vi "HFRR ADV v06 new software.vi"() -> ()   [LabVIEW 2025] (continued)
                  n3117 = local write "S 59"(w4151) -> ()
                }
                frame 59 {
                  n3118 = local write "S 60"(w4152) -> ()
                }
                frame 60 {
                  n3119 = local write "S 62"(w4153) -> ()
                }
                frame 61 {
                  n3120 = local write "S 63"(w4154) -> ()
                }
                frame 62 {
                  n3121 = local write "S 64"(w4155) -> ()
                }
                frame 63 {
                  n3122 = local write "S 65"(w4156) -> ()
                }
                frame 64 {
                  n3123 = local write "S 66"(w4157) -> ()
                }
                frame 65 {
                  n3124 = local write "S 67"(w4158) -> ()
                }
                frame 66 {
                  n3125 = local write "S 68"(w4159) -> ()
                }
                frame 67 {
                  n3126 = local write "S 69"(w4160) -> ()
                }
                frame 68 {
                  n3127 = local write "S 70"(w4161) -> ()
                }
                frame 69 {
                  n3128 = local write "S 71"(w4162) -> ()
                }
                frame 70 {
                  n3129 = local write "S 72"(w4163) -> ()
                }
                frame 71 {
                  n3130 = local write "S 73"(w4164) -> ()
                }
                frame 72 {
                  n3131 = local write "S 74"(w4165) -> ()
                }
                frame 73 {
                  n3132 = local write "S 75"(w4166) -> ()
                }
                frame 74 {
                  n3133 = local write "S 76"(w4167) -> ()
                }
                frame 75 {
                  n3134 = local write "S 77"(w4168) -> ()
                }
                frame 76 {
                  n3135 = local write "S 78"(w4169) -> ()
                }
                frame 77 {
                  n3136 = local write "S 79"(w4170) -> ()
                }
                frame 79 {
                  n3137 = property on="Sample Temperature ( °C )" class="XYGraph (strict)"("Y Scale.Name Label.Text"=w4171) -> ()  [unwired: 2 in, 2 out]
                }
                frame 80 {
                  n3138 = local write "S 81"(w4172) -> ()
                  n3139 = property on="Humidity ( %RH )" class="XYGraph (strict)"("Y Scale.Name Label.Text"=w4172) -> ()  [unwired: 2 in, 2 out]
                }
                frame 78 {
                  n3140 = property on="Air Temperature  ( °C )" class="XYGraph (strict)"("X Scale.Name Label.Text"=w4173) -> ()  [unwired: 2 in, 2 out]
                  n3141 = property on="Humidity ( %RH )" class="XYGraph (strict)"("X Scale.Name Label.Text"=w4173) -> ()  [unwired: 2 in, 2 out]
                  n3142 = property on="Sample Temperature ( °C )" class="XYGraph (strict)"("X Scale.Name Label.Text"=w4173) -> ()  [unwired: 2 in, 2 out]
                  n3143 = property on="Coefficient Of Friction" class="XYGraph (strict)"("X Scale.Name Label.Text"=w4173) -> ()  [unwired: 2 in, 2 out]
                }
                frame 81 {
                  n3144 = property on="Air Temperature  ( °C )" class="XYGraph (strict)"("Y Scale.Name Label.Text"=w4174) -> ()  [unwired: 2 in, 2 out]
                }
                frame 82 {
                  n3145 = local write "S 84"(w4175) -> ()
                }
                frame 83 {
                  n3146 = local write "S 85"(w4176) -> ()
                }
                frame 84 {
                  n3147 = local write "S 86"(w4177) -> ()
                }
                frame 85 {
                  n3148 = local write "S 87"(w4178) -> ()
                }
                frame 86 {
                  n3149 = local write "S 88"(w4179) -> ()
                }
                frame 87 {
                }
                frame 88 {
                  n3150 = local write "S 90"(w4181) -> ()
                }
                frame 89 {
                  n3151 = local write "S 91"(w4182) -> ()
                }
                frame 90 {
                  n3152 = local write "S 92"(w4183) -> ()
                }
                frame 91 {
                  n3153 = local write "S 93"(w4184) -> ()
                }
                frame 92 {
                  n3154 = local write "S 94"(w4185) -> ()
                }
                frame 93 {
                  n3155 = local write "S 95"(w4186) -> ()
                }
                frame 94 {
                  n3156 = local write "S 96"(w4187) -> ()
                }
                frame 95 {
                  n3157 = local write "S 97"(w4188) -> ()
                }
                frame 96 {
                  n3158 = local write "S 98"(w4189) -> ()
                }
                frame 97 {
                  n3159 = local write "S 99"(w4190) -> ()
                }
                frame 98 {
                  n3160 = local write "S 100"(w4191) -> ()
                }
                frame 99 {
                  n3161 = local write "S 101"(w4192) -> ()
                }
                frame 100 {
                  n3162 = local write "S 102"(w4193) -> ()
                }
                frame 101 {
                  n3163 = local write "S 103"(w4194) -> ()
                }
                frame 102 {
                  n3164 = local write "S 104"(w4195) -> ()
                }
                frame 103 {
                  n3165 = local write "S 105"(w4196) -> ()
                }
                frame 104 {
                  n3166 = local write "S 106"(w4197) -> ()
                }
                frame 105 {
                }
                frame 106 {
                  n3167 = property on="OK Button 17" class="Bool (strict)"("Boolean Text.Text"=w4198) -> ()  [unwired: 2 in, 2 out]
                }
                frame 107 {
                  n3168 = property on="OK Button 16" class="Bool (strict)"("Boolean Text.Text"=w4199) -> ()  [unwired: 2 in, 2 out]
                }
                frame 108 {
                  n3169 = property on="TITTLE" class="Str"("Caption.Text"=w4200) -> ()  [unwired: 2 in, 2 out]
                }
                frame 109 {
                  "String 30" <- w4201
                }
                frame 110 {
                  n3170 = property on="Test Date" class="Str"("Caption.Text"=w4202) -> ()  [unwired: 2 in, 2 out]
                  "String 31" <- w4202
                }
                frame 111 {
                  n3171 = property on="Sample ID" class="Str"("Caption.Text"=w4203) -> ()  [unwired: 2 in, 2 out]
                  "String 32" <- w4203
                }
                frame 112 {
                  n3172 = property on="Tested by" class="Str"("Caption.Text"=w4204) -> ()  [unwired: 2 in, 2 out]
                  "String 33" <- w4204
                }
                frame 113 {
                  n3173 = property on="System Configured Printers 2" class="Arr (strict)"("Caption.Text"=w4205) -> ()  [unwired: 2 in, 2 out]
                }
                frame 114 {
                  n3174 = property on="Selected Printer" class="Str"("Caption.Text"=w4206) -> ()  [unwired: 2 in, 2 out]
                }
                frame 115 {
                  n3175 = property on="Select Printer 3" class="DigNum (strict)"("Caption.Text"=w4207) -> ()  [unwired: 2 in, 2 out]
                }
                frame 116 {
                  n3176 = property on="Print" class="Bool (strict)"("Boolean Text.Text"=w4208) -> ()  [unwired: 2 in, 2 out]
                }
                frame 117 {
                  "String 41" <- w4209
                }
                frame 118 {
                  n3177 = property on="tested by" class="Str"("Caption.Text"=w4210) -> ()  [unwired: 2 in, 2 out]
                }
                frame 119 {
                }
                frame 120 {
                  n3178 = property on="Export" class="Bool (strict)"("Boolean Text.Text"=w4211) -> ()  [unwired: 2 in, 2 out]
                }
                frame 121 {
                  n3179 = property on="TEMP INTERCEPT:" class="DigNum (strict)"("Caption.Text"=w4212) -> ()  [unwired: 2 in, 2 out]
                }
                frame 122 {
                  n3180 = property on="AIR TEMP INTERCEPT:" class="DigNum (strict)"("Caption.Text"=w4213) -> ()  [unwired: 2 in, 2 out]
                }
                frame 123 {
                  n3181 = property on="Select File Type" class="Enum (strict)"("Caption.Text"=w4214) -> ()  [unwired: 2 in, 2 out]
                }
                frame 124 {
                  n3182 = property on="s.NO" class="Str"("Caption.Text"=w4215) -> ()  [unwired: 2 in, 2 out]
                  "String 45" <- w4215
                }
                frame 125 {
                  n3183 = property on="trip1 8" class="Bool (strict)"("Boolean Text.Text"=w4216) -> ()  [unwired: 2 in, 2 out]
                }
                frame 126, Default {
                }
              }
            }
          }
          frame #1 {
            w4224 = TRUE ("Visible")
            n3184 = local read "S 91"() -> (w4241:string)
            n3185 = local read "S 90"() -> (w4240:string)
            n3186 = local read "S 88"() -> (w4239:string)
            n3187 = property on="File Path" class="Path"("Caption.Text"=w4240) -> ()  [unwired: 2 in, 2 out]
            n3188 = property on="SrvM CP" class="Bool (strict)"("Boolean Text.Text"=w4239) -> ()  [unwired: 2 in, 2 out]
            n3189 = local read "S 71"() -> (w4234:string)
            n3190 = local read "S 86"() -> (w4236:string)
            n3191 = local read "S 85"() -> (w4237:string)
            n3192 = local read "S 87"() -> (w4235:string)
            n3193 = local read "S 84"() -> (w4238:string)
            n3194 = local read "S 103"() -> (w4223:string)
            n3195 = local read "S 104"() -> (w4222:string)
            n3196 = property on="ENTER THE NEW PASSWORD" class="Str"("Caption.Text"=w4235) -> ()  [unwired: 2 in, 2 out]
            n3197 = property on="Password" class="Str"("Caption.Text"=w4237) -> ()  [unwired: 2 in, 2 out]
            n3198 = property on="ENTER CURRENT PASSWORD" class="Str"("Caption.Text"=w4236) -> ()  [unwired: 2 in, 2 out]
            n3199 = property on="EDIT" class="Bool (strict)"("Boolean Text.Text"=w4234) -> ()  [unwired: 2 in, 2 out]
            n3200 = property on="SAVE" class="Bool (strict)"("Boolean Text.Text"=w4238) -> ()  [unwired: 2 in, 2 out]
            n3201 = Build Array(w4223, w4222) -> (w4221:string[])
            n3202 = property on="Heater Button" class="Bool (strict)"("Strings [4]"=w4221) -> ()  [unwired: 2 in, 2 out]
            n3203 = property on="CH-HUMIDITY WET" class="DigNum (strict)"("Caption.Size to Text?"=w4224) -> ()  [unwired: 2 in, 2 out]
            n3204 = property on="CH-HUMIDITY DRY" class="DigNum (strict)"("Caption.Size to Text?"=w4224) -> ()  [unwired: 2 in, 2 out]
            n3205 = property on="CH-POWER -" class="DigNum (strict)"("Caption.Size to Text?"=w4224) -> ()  [unwired: 2 in, 2 out]
            n3206 = property on="CH-HEATER" class="DigNum (strict)"("Caption.Size to Text?"=w4224) -> ()  [unwired: 2 in, 2 out]
            n3207 = property on="CH-POWER +" class="DigNum (strict)"("Caption.Size to Text?"=w4224) -> ()  [unwired: 2 in, 2 out]
            n3208 = local read "S 92"() -> (w4233:string)
            n3209 = local read "S 93"() -> (w4232:string)
            n3210 = local read "S 105"() -> (w4219:string)
            n3211 = local read "S 106"() -> (w4218:string)
            n3212 = Build Array(w4233, w4232) -> ()  [unwired: 1 out]
            n3213 = Build Array(w4219, w4218) -> (w4220:string[])
            n3214 = local read "S 95"() -> (w4230:string)
            n3215 = local read "S 94"() -> (w4231:string)
            n3216 = local read "bs"() -> (w4246:string)
            n3217 = local read "as"() -> (w4247:string)
            n3218 = property on="Humidity" class="Bool (strict)"("Strings [4]"=w4220) -> ()  [unwired: 2 in, 2 out]
            n3219 = Concatenate Strings(w4246, "\r", w4247) -> ()  [unwired: 1 out]
            n3220 = property on="STROKE GAIN :" class="DigNum (strict)"("Caption.Text"=w4230) -> ()  [unwired: 2 in, 2 out]
            n3221 = property on="DISPLACEMENT :" class="DigNum (strict)"("Caption.Text"=w4231) -> ()  [unwired: 2 in, 2 out]
            n3222 = property on="Rh After" class="DigNum (strict)"("Caption.Size to Text?"=TRUE ("Caption.Size to Text")) -> ()  [unwired: 2 in, 2 out]
            n3223 = local read "S 48"() -> (w4270:string)
            n3224 = local read "S 50"() -> (w4268:string)
            n3225 = local read "S 51"() -> (w4267:string)
            n3226 = local read "S 49"() -> (w4269:string)
            n3227 = local read "S 52"() -> (w4266:string)
            n3228 = local read "as"() -> (w4251:string)
            n3229 = local read "bs"() -> (w4252:string)
            n3230 = local read "S 56"() -> (w4265:string)
            n3231 = local read "S 57"() -> (w4264:string)
            n3232 = local read "S 58"() -> (w4263:string)
            n3233 = local read "S 59"() -> (w4262:string)
            n3234 = property on="OPEN" class="Bool (strict)"("Boolean Text.Text"=w4266) -> ()  [unwired: 2 in, 2 out]
            n3235 = property on="OPEN 1" class="Bool (strict)"("Boolean Text.Text"=w4270) -> ()  [unwired: 2 in, 2 out]
            n3236 = property on="OPEN 2" class="Bool (strict)"("Boolean Text.Text"=w4269) -> ()  [unwired: 2 in, 2 out]
            n3237 = property on="OPEN 3" class="Bool (strict)"("Boolean Text.Text"=w4268) -> ()  [unwired: 2 in, 2 out]
            n3238 = property on="OPEN 4" class="Bool (strict)"("Boolean Text.Text"=w4267) -> ()  [unwired: 2 in, 2 out]
            n3239 = Concatenate Strings(w4252, "\r", w4251) -> ()  [unwired: 1 out]
            n3240 = local read "S 102"() -> (w4225:string)
            n3241 = property on="КОФ1" class="DigNum (strict)"("Caption.Text"=w4265) -> ()  [unwired: 2 in, 2 out]
            n3242 = local read "S 98"() -> (w4229:string)
            n3243 = local read "S 99"() -> (w4228:string)
            n3244 = local read "S 100"() -> (w4227:string)
            n3245 = local read "S 101"() -> (w4226:string)
            n3246 = property on="КОФ2" class="DigNum (strict)"("Caption.Text"=w4264) -> ()  [unwired: 2 in, 2 out]
            n3247 = property on="КОФ3" class="DigNum (strict)"("Caption.Text"=w4263) -> ()  [unwired: 2 in, 2 out]
            n3248 = property on="КОФ4" class="DigNum (strict)"("Caption.Text"=w4262) -> ()  [unwired: 2 in, 2 out]
            n3249 = local read "bs"() -> (w4250:string)
            n3250 = local read "as"() -> (w4249:string)
            n3251 = property on="CH-POWER +" class="DigNum (strict)"("Caption.Text"=w4229) -> ()  [unwired: 2 in, 2 out]
            n3252 = property on="CH-POWER -" class="DigNum (strict)"("Caption.Text"=w4228) -> ()  [unwired: 2 in, 2 out]
            n3253 = property on="CH-HEATER" class="DigNum (strict)"("Caption.Text"=w4227) -> ()  [unwired: 2 in, 2 out]
            n3254 = property on="CH-HUMIDITY DRY" class="DigNum (strict)"("Caption.Text"=w4226) -> ()  [unwired: 2 in, 2 out]
            n3255 = property on="CH-HUMIDITY WET" class="DigNum (strict)"("Caption.Text"=w4225) -> ()  [unwired: 2 in, 2 out]
            n3256 = local read "S 60"() -> (w4261:string)
            n3257 = local read "S 54"() -> (w4271:string)
            n3258 = Concatenate Strings(w4250, "\r", w4249) -> ()  [unwired: 1 out]
            n3259 = Concatenate Strings(w4271, w4261) -> ()  [unwired: 1 out]
            n3260 = local read "S 77"() -> (→"String 43":string)
            n3261 = local read "S 76"() -> (w4244:string)
            n3262 = local read "S 78"() -> (w4243:string)
            n3263 = local read "S 71"() -> (w4255:string)
            n3264 = local read "S 66"() -> (w4260:string)
            n3265 = local read "S 67"() -> (w4259:string)
            n3266 = local read "S 68"() -> (w4258:string)
            n3267 = local read "S 69"() -> (w4257:string)
            n3268 = local read "S 70"() -> (w4256:string)
            n3269 = property on="AIR TEMP" class="DigNum (strict)"("Caption.Text"=w4243) -> ()  [unwired: 2 in, 2 out]
            n3270 = property on="Set Strk" class="DigNum (strict)"("Caption.Text"=w4244) -> ()  [unwired: 2 in, 2 out]
            n3271 = property on="FRIC. FORCE :" class="DigNum (strict)"("Caption.Text"=w4260) -> ()  [unwired: 2 in, 2 out]
            n3272 = property on="TEMPERATURE :" class="DigNum (strict)"("Caption.Text"=w4259) -> ()  [unwired: 2 in, 2 out]
            n3273 = property on="SPEED OUT:" class="DigNum (strict)"("Caption.Text"=w4258) -> ()  [unwired: 2 in, 2 out]
            n3274 = property on="AIR TEMPERATURE :" class="DigNum (strict)"("Caption.Text"=w4257) -> ()  [unwired: 2 in, 2 out]
            n3275 = property on="HUMIDITY:" class="DigNum (strict)"("Caption.Text"=w4256) -> ()  [unwired: 2 in, 2 out]
            n3276 = property on="EDIT" class="Bool (strict)"("Boolean Text.Text"=w4255) -> ()  [unwired: 2 in, 2 out]
            n3277 = local read "S 79"() -> (w4242:string)
          }
          frame #2 {
          }
        }
        n3278 = local write "Lan flag"(10.0 ("Lan flag")) -> ()
      }
      frame Enabled {
      }
    }
    n3279 = Wait (ms)(milliseconds to wait=u32 2000) -> ()  [unwired: 1 out]
    n3280 = local read "Quit"() -> (w4045:bool)
  }
  n3281 = disable-structure shown="Disabled" {
    frame Disabled {
      n3282 = while {
        tunnel: [w4273] -> _
        i -> [w4273]
        stop <- w4272 continue-if-true
        n3283 = Wait (ms)(milliseconds to wait=u32 50) -> ()  [unwired: 1 out]
        n3284 = stacked-sequence {
          frame #0 {
            # "Controls Text color"
            # "Controls BG color"
            n3285 = property on="FILE" class="Str"("Text.Text Colors:Text Color"="SC  Text") -> ()  [unwired: 2 in, 2 out]
            n3286 = property on="Fuel Discription :" class="Str"("Text.Text Colors:Text Color"="SC  Text") -> ()  [unwired: 2 in, 2 out]
            n3287 = property on="tested by" class="Str"("Text.Text Colors:Text Color"="SC  Text") -> ()  [unwired: 2 in, 2 out]
            n3288 = property on="Remarks :" class="Str"("Text.Text Colors:Text Color"="SC  Text") -> ()  [unwired: 2 in, 2 out]
            n3289 = property class="DigNum (strict)"("Numeric Text.Text Colors:BG Color"="NC BG") -> ()  [unwired: 2 in, 2 out]
            n3290 = property class="DigNum (strict)"("Numeric Text.Text Colors:BG Color"="NC BG") -> ()  [unwired: 2 in, 2 out]
            n3291 = property class="DigNum (strict)"("Numeric Text.Text Colors:BG Color"="NC BG") -> ()  [unwired: 2 in, 2 out]
            n3292 = property class="DigNum (strict)"("Numeric Text.Text Colors:BG Color"="NC BG") -> ()  [unwired: 2 in, 2 out]
            n3293 = property class="DigNum (strict)"("Numeric Text.Text Colors:BG Color"="NC BG") -> ()  [unwired: 2 in, 2 out]
            n3294 = property class="DigNum (strict)"("Numeric Text.Text Colors:BG Color"="NC BG") -> ()  [unwired: 2 in, 2 out]
            n3295 = property class="DigNum (strict)"("Numeric Text.Text Colors:BG Color"="NC BG") -> ()  [unwired: 2 in, 2 out]
            n3296 = property class="DigNum (strict)"("Numeric Text.Text Colors:BG Color"="NC BG") -> ()  [unwired: 2 in, 2 out]
            n3297 = property class="DigNum (strict)"("Numeric Text.Text Colors:BG Color"="NC BG") -> ()  [unwired: 2 in, 2 out]
            n3298 = property class="DigNum (strict)"("Numeric Text.Text Colors:BG Color"="NC BG") -> ()  [unwired: 2 in, 2 out]
            n3299 = property class="DigNum (strict)"("Numeric Text.Text Colors:BG Color"="NC BG") -> ()  [unwired: 2 in, 2 out]
            n3300 = property class="DigNum (strict)"("Numeric Text.Text Colors:BG Color"="NC BG") -> ()  [unwired: 2 in, 2 out]
            n3301 = property on="FILE" class="Str"("Text.Text Colors:BG Color"="SC BG 3") -> ()  [unwired: 2 in, 2 out]
            n3302 = property on="Fuel Discription :" class="Str"("Text.Text Colors:BG Color"="SC BG 3") -> ()  [unwired: 2 in, 2 out]
            n3303 = property on="tested by" class="Str"("Text.Text Colors:BG Color"="SC BG 3") -> ()  [unwired: 2 in, 2 out]
            n3304 = property on="Remarks :" class="Str"("Text.Text Colors:BG Color"="SC BG 3") -> ()  [unwired: 2 in, 2 out]
            n3305 = property class="DigNum (strict)"("Numeric Text.Text Colors:Text Color"="NC Text") -> ()  [unwired: 2 in, 2 out]
            n3306 = property class="DigNum (strict)"("Numeric Text.Text Colors:Text Color"="NC Text") -> ()  [unwired: 2 in, 2 out]
            n3307 = property class="DigNum (strict)"("Numeric Text.Text Colors:Text Color"="NC Text") -> ()  [unwired: 2 in, 2 out]
            n3308 = property class="DigNum (strict)"("Numeric Text.Text Colors:Text Color"="NC Text") -> ()  [unwired: 2 in, 2 out]
            n3309 = property class="DigNum (strict)"("Numeric Text.Text Colors:Text Color"="NC Text") -> ()  [unwired: 2 in, 2 out]
            n3310 = property class="DigNum (strict)"("Numeric Text.Text Colors:Text Color"="NC Text") -> ()  [unwired: 2 in, 2 out]
            n3311 = property class="DigNum (strict)"("Numeric Text.Text Colors:Text Color"="NC Text") -> ()  [unwired: 2 in, 2 out]
            n3312 = property class="DigNum (strict)"("Numeric Text.Text Colors:Text Color"="NC Text") -> ()  [unwired: 2 in, 2 out]
            n3313 = property class="DigNum (strict)"("Numeric Text.Text Colors:Text Color"="NC Text") -> ()  [unwired: 2 in, 2 out]
            n3314 = property class="DigNum (strict)"("Numeric Text.Text Colors:Text Color"="NC Text") -> ()  [unwired: 2 in, 2 out]
            n3315 = property class="DigNum (strict)"("Numeric Text.Text Colors:Text Color"="NC Text") -> ()  [unwired: 2 in, 2 out]
            n3316 = property class="DigNum (strict)"("Numeric Text.Text Colors:Text Color"="NC Text") -> ()  [unwired: 2 in, 2 out]
            n3317 = property class="DigNum (strict)"("Numeric Text.Text Colors:Text Color"="NI Text  2") -> ()  [unwired: 2 in, 2 out]
            n3318 = property class="DigNum (strict)"("Numeric Text.Text Colors:Text Color"="NI Text  2") -> ()  [unwired: 2 in, 2 out]
            n3319 = property class="DigNum (strict)"("Numeric Text.Text Colors:Text Color"="NI Text  2") -> ()  [unwired: 2 in, 2 out]
            n3320 = property class="DigNum (strict)"("Numeric Text.Text Colors:Text Color"="NI Text  2") -> ()  [unwired: 2 in, 2 out]
            n3321 = property class="DigNum (strict)"("Numeric Text.Text Colors:Text Color"="NI Text  2") -> ()  [unwired: 2 in, 2 out]
            n3322 = property class="DigNum (strict)"("Numeric Text.Text Colors:Text Color"="NI Text  2") -> ()  [unwired: 2 in, 2 out]
            n3323 = property class="DigNum (strict)"("Numeric Text.Text Colors:Text Color"="NI Text  2") -> ()  [unwired: 2 in, 2 out]
            n3324 = property class="DigNum (strict)"("Numeric Text.Text Colors:Text Color"="NI Text  2") -> ()  [unwired: 2 in, 2 out]
            n3325 = property class="DigNum (strict)"("Numeric Text.Text Colors:Text Color"="NI Text  2") -> ()  [unwired: 2 in, 2 out]
            n3326 = property class="DigNum (strict)"("Numeric Text.Text Colors:Text Color"="NI Text  2") -> ()  [unwired: 2 in, 2 out]
            n3327 = property class="DigNum (strict)"("Numeric Text.Text Colors:Text Color"="NI Text  2") -> ()  [unwired: 2 in, 2 out]
            n3328 = property class="DigNum (strict)"("Numeric Text.Text Colors:Text Color"="NI Text  2") -> ()  [unwired: 2 in, 2 out]
            n3329 = property class="DigNum (strict)"("Numeric Text.Text Colors:Text Color"="NI Text  2") -> ()  [unwired: 2 in, 2 out]
            n3330 = property class="DigNum (strict)"("Numeric Text.Text Colors:Text Color"="NI Text  2") -> ()  [unwired: 2 in, 2 out]
            n3331 = property class="DigNum (strict)"("Numeric Text.Text Colors:Text Color"="NI Text  2") -> ()  [unwired: 2 in, 2 out]
            n3332 = property on="Coefficient Of Friction" class="XYGraph (strict)"("Plot Area:Colors:FG Color"="GFG  2", "Plot Area:Colors:BG Color"="GBG   2") -> ()  [unwired: 2 in, 2 out]
            n3333 = property on="Humidity ( %RH )" class="XYGraph (strict)"("Plot Area:Colors:FG Color"="GFG  2", "Plot Area:Colors:BG Color"="GBG   2") -> ()  [unwired: 2 in, 2 out]
            n3334 = property on="Air Temperature  ( °C )" class="XYGraph (strict)"("Plot Area:Colors:FG Color"="GFG  2", "Plot Area:Colors:BG Color"="GBG   2") -> ()  [unwired: 2 in, 2 out]
            n3335 = property on="Sample Temperature ( °C )" class="XYGraph (strict)"("Plot Area:Colors:FG Color"="GFG  2", "Plot Area:Colors:BG Color"="GBG   2") -> ()  [unwired: 2 in, 2 out]
            n3336 = property class="DigNum (strict)"("Numeric Text.Text Colors:BG Color"="NI BG 2") -> ()  [unwired: 2 in, 2 out]
            n3337 = property class="DigNum (strict)"("Numeric Text.Text Colors:BG Color"="NI BG 2") -> ()  [unwired: 2 in, 2 out]
            n3338 = property class="DigNum (strict)"("Numeric Text.Text Colors:BG Color"="NI BG 2") -> ()  [unwired: 2 in, 2 out]
            n3339 = property class="DigNum (strict)"("Numeric Text.Text Colors:BG Color"="NI BG 2") -> ()  [unwired: 2 in, 2 out]
            n3340 = property class="DigNum (strict)"("Numeric Text.Text Colors:BG Color"="NI BG 2") -> ()  [unwired: 2 in, 2 out]
            n3341 = property class="DigNum (strict)"("Numeric Text.Text Colors:BG Color"="NI BG 2") -> ()  [unwired: 2 in, 2 out]
            n3342 = property class="DigNum (strict)"("Numeric Text.Text Colors:BG Color"="NI BG 2") -> ()  [unwired: 2 in, 2 out]
            n3343 = property class="DigNum (strict)"("Numeric Text.Text Colors:BG Color"="NI BG 2") -> ()  [unwired: 2 in, 2 out]
            n3344 = property class="DigNum (strict)"("Numeric Text.Text Colors:BG Color"="NI BG 2") -> ()  [unwired: 2 in, 2 out]
            n3345 = property class="DigNum (strict)"("Numeric Text.Text Colors:BG Color"="NI BG 2") -> ()  [unwired: 2 in, 2 out]
            n3346 = property class="DigNum (strict)"("Numeric Text.Text Colors:BG Color"="NI BG 2") -> ()  [unwired: 2 in, 2 out]
            n3347 = property class="DigNum (strict)"("Numeric Text.Text Colors:BG Color"="NI BG 2") -> ()  [unwired: 2 in, 2 out]
            n3348 = property class="DigNum (strict)"("Numeric Text.Text Colors:BG Color"="NI BG 2") -> ()  [unwired: 2 in, 2 out]
            n3349 = property class="DigNum (strict)"("Numeric Text.Text Colors:BG Color"="NI BG 2") -> ()  [unwired: 2 in, 2 out]
            n3350 = property class="DigNum (strict)"("Numeric Text.Text Colors:BG Color"="NI BG 2") -> ()  [unwired: 2 in, 2 out]
            n3351 = property class="Bool"("Colors [4]"="Boolean BC T & BG") -> ()  [unwired: 2 in, 2 out]
            n3352 = property on="Save & Continue" class="Bool (strict)"("Colors [4]"="Boolean BC T & BG") -> ()  [unwired: 2 in, 2 out]
            n3353 = property on="Heater Button" class="Bool (strict)"("Colors [4]"="Boolean BC T & BG") -> ()  [unwired: 2 in, 2 out]
            n3354 = property class="Bool"("Colors [4]"="Boolean BC T & BG") -> ()  [unwired: 2 in, 2 out]
            n3355 = property on="Humidity" class="Bool (strict)"("Colors [4]"="Boolean BC T & BG") -> ()  [unwired: 2 in, 2 out]
            n3356 = property class="Bool (strict)"("Colors [4]"="Boolean BC T & BG") -> ()  [unwired: 2 in, 2 out]
            n3357 = property on="RUN" class="Bool (strict)"("Colors [4]"="Boolean BC T & BG") -> ()  [unwired: 2 in, 2 out]
            n3358 = property on="trip1 8" class="Bool (strict)"("Colors [4]"="Boolean BC T & BG") -> ()  [unwired: 2 in, 2 out]
            n3359 = property class="Bool"("Colors [4]"="Boolean BC T & BG") -> ()  [unwired: 2 in, 2 out]
            n3360 = property class="Bool (strict)"("Colors [4]"="Boolean BC T & BG") -> ()  [unwired: 2 in, 2 out]
            n3361 = property on="OPEN 1" class="Bool (strict)"("Colors [4]"="Boolean BC T & BG 2") -> ()  [unwired: 2 in, 2 out]
            n3362 = property on="OPEN 2" class="Bool (strict)"("Colors [4]"="Boolean BC T & BG 2") -> ()  [unwired: 2 in, 2 out]
            n3363 = property on="OPEN 3" class="Bool (strict)"("Colors [4]"="Boolean BC T & BG 2") -> ()  [unwired: 2 in, 2 out]
            n3364 = property on="OPEN 4" class="Bool (strict)"("Colors [4]"="Boolean BC T & BG 2") -> ()  [unwired: 2 in, 2 out]
            n3365 = property on="OPEN" class="Bool (strict)"("Colors [4]"="Boolean BC T & BG 2") -> ()  [unwired: 2 in, 2 out]
            n3366 = property on="rstv2" class="Bool"("Colors [4]"="Boolean BC T & BG 2") -> ()  [unwired: 2 in, 2 out]
            n3367 = property on="RST CP" class="Bool"("Colors [4]"="Boolean BC T & BG 2") -> ()  [unwired: 2 in, 2 out]
            n3368 = property on="RSTV1 3" class="Bool"("Colors [4]"="Boolean BC T & BG 2") -> ()  [unwired: 2 in, 2 out]
            n3369 = property on="RSTV1 2" class="Bool"("Colors [4]"="Boolean BC T & BG 2") -> ()  [unwired: 2 in, 2 out]
          }
          frame #1 {
          }
        }
        n3370 = local read "Quit"() -> (w4272:bool)
      }
    }
    frame Enabled {
    }
  }
  n3371 = while {
    shift-right: [w4290] -> _
    shift-left: _ -> [w4291]
    shift-right: [w4288] -> _
    shift-left: T14 {"Read Heave and Surge"="", "Bytes at Heave Port"=0.0, "Heave and Surge COM Port:"="COM9", "Com Port 2"="COM7", "Residual Due"="", "Heave COM Status 2"=TRUE, "Heave COM Status"=TRUE, "Port 2"=TRUE, "Sway PPR"=6400.0, "Surge PPR"=6400.0, "Heave PPR"=6400.0, "Sway Pitch"=2.0, "Surge Pitch"=3.0, "Heave Pitch"=4.0, "Sway Pulses/mm"=320.0, "Surge Pulses/mm"=1600.0, "Heave Pulses/mm"=1600.0, "inner loop"=0.0, "Read Heave and Surge 2"="", "String 36"="", "Write S"=FALSE, "WriteCC1"=[""], "Heave COM Loop"=0, "LastCom"="", "EXIT"=FALSE, "Error Heave"={"status"=TRUE, "code"=-1073807343, "source"=""}} -> [w4287]
    shift-right: [w4285] -> _
    shift-left: enum16{"init", "MAIN", "Panel Close"}."init" -> [w4286]
    stop <- w4289 stop-if-true
    n3372 = case shown="\"init\"" w4286 {
      tunnel: w4291 -> [w4305 w4320 w4390 w4392]
      tunnel: [w4299 w4338 w4390 w4392] -> w4290
      tunnel: [_ _ TRUE _] -> w4289
      tunnel: [w4295 w4335 w4388 w4391] -> w4288
      tunnel: w4287 -> [w4302 w4319 w4388 w4391]
      tunnel: [enum16{"init", "MAIN", "Panel Close"}."MAIN" w4313 _ _] -> w4285
      frame "init" {
        n3373 = Bundle By Name(cluster=w4302, "Heave and Surge COM Port:"="C3 :") -> (w4301:T14)
        n3374 = call "Instrument fgv.vi"("Enum"=T26."INIT", "error in (no error) 2"=w4305, "INPUT"=w4301) -> ("error"=w4303:errorcluster, "output"=w4298:T14)  [unwired: 6 in, 1 out]
        n3375 = case shown="No Error" w4303 {
          selector: w4303 -> [w4307 _]
          tunnel: [w4307 w4311] -> w4299
          tunnel: w4298 -> [w4306 w4309]
          tunnel: [w4306 w4308] -> w4296
          frame No Error {
          }
          frame Error {
            n3376 = call "Instrument fgv.vi"("Enum"=T26."ERROR INIT", "INPUT"=w4309) -> ("error"=w4312:errorcluster, "output"=w4308:T14)  [unwired: 7 in, 1 out]
            n3377 = call <vilib>:"Clear Errors.vi"("error in (no error)"=w4312) -> ("error out"=w4311:errorcluster)  [unwired: 5 in, 1 out]
          }
        }
        n3378 = local read "LastCom"() -> (w4294:string)
        n3379 = Unbundle By Name(w4296) -> ("Heave COM Status 2"=→"COM Status" →"Instrument Status":bool, "Error Heave"=→"Error":errorcluster)  [unwired: 1 out]
        n3380 = Bundle By Name(cluster=w4296, "LastCom"=w4294) -> (w4295:T14)
      }
      frame "MAIN" {
        n3381 = Unbundle By Name(w4319) -> ("Com Port 2"=w4340:refnum<visa-resource-name>)
        n3382 = local write "Com Port 4"(w4340) -> ()
        n3383 = local read "C3 :"() -> (w4317:refnum<visa-resource-name>)
        n3384 = Divide(x="Heave PPR", y="Heave Pitch") -> (x/y=→"Heave Pulses/mm":dbl)
        n3385 = Bundle By Name(cluster=w4319, "Heave and Surge COM Port:"=w4317) -> (w4318:T14)
        n3386 = Equal?(x=w4340, y=w4317) -> (x = y?=w4339:bool)
        n3387 = Divide(x="Sway PPR", y="Sway Pitch") -> (x/y=→"Sway Pulses/mm":dbl)
        n3388 = case shown="False" w4339 {
          tunnel: [w4344 w4361] -> w4338
          tunnel: w4320 -> [w4345 w4367]
          tunnel: w4318 -> [w4343 w4365]
          tunnel: [w4342 w4360] -> w4335
          frame False {
            n3389 = call <vilib>:"Clear Errors.vi"("error in (no error)"=w4345) -> ("error out"=w4341:errorcluster)  [unwired: 5 in, 1 out]
            n3390 = call "Instrument fgv.vi"("Enum"=T26."ERROR INIT", "error in (no error) 2"=w4341, "INPUT"=w4343) -> ("error"=w4347:errorcluster, "output"=w4342:T14)  [unwired: 6 in, 1 out]
            n3391 = call <vilib>:"Clear Errors.vi"("error in (no error)"=w4347) -> ("error out"=w4344:errorcluster)  [unwired: 5 in, 1 out]
          }
          frame True {
            n3392 = call "Instrument fgv.vi"("Enum"=T26."READ", "error in (no error) 2"=w4367, "INPUT"=w4365) -> ("error"=w4366:errorcluster, "output"=w4357:T14)  [unwired: 6 in, 1 out]
            n3393 = Bundle By Name(cluster=w4357, "String 36"="String 11") -> (w4356:T14)
            n3394 = case shown="True" "Write S" {
              selector: "Write S" -> [_ w4387]
              tunnel: w4366 -> [w4380 w4386]
              tunnel: [w4380 w4385] -> w4353
              tunnel: w4356 -> [w4379 w4382]
              tunnel: [w4379 w4381] -> w4352
              frame False {
              }
              frame True {
                n3395 = Not(x=w4387) -> (.not. x?=w4383:bool)
                n3396 = local write "Write S"(w4383) -> ()
                n3397 = call "Instrument fgv.vi"("Enum"=T26."MANUAL WRITE", "error in (no error) 2"=w4386, "INPUT"=w4382) -> ("error"=w4385:errorcluster, "output"=w4381:T14)  [unwired: 6 in, 1 out]
              }
            }
            n3398 = Array Size(array="WriteHumidity") -> (size(s)=w4350:i32)
            n3399 = Greater Than 0?(x=w4350) -> (x > 0?=w4348:bool)
            n3400 = call "Instrument fgv.vi"("Enum"=T26."WRITE", "error in (no error) 2"=w4353, "WriteCC1"="WriteHumidity", "INPUT"=w4352) -> ("error"=w4363:errorcluster, "WriteCC1 2"=w4351:string[], "output"=w4362:T14)  [unwired: 5 in]
            n3401 = case shown="True" w4348 {
              tunnel: w4351 -> [_ w4369]
              frame False {
              }
              frame True {
                n3402 = local write "WriteHumidity"(w4369) -> ()
              }
            }
            n3403 = case shown="Error" w4363 {
              selector: w4363 -> [w4370 w4373]
              tunnel: w4362 -> [w4371 w4378]
              tunnel: [w4371 w4377] -> w4360
              tunnel: [w4370 w4375] -> w4361
              frame No Error {
              }
              frame Error {
                n3404 = call <vilib>:"Clear Errors.vi"("error in (no error)"=w4373) -> ("error out"=w4372:errorcluster)  [unwired: 5 in, 1 out]
                n3405 = call "Instrument fgv.vi"("Enum"=T26."ERROR INIT", "error in (no error) 2"=w4372, "INPUT"=w4378) -> ("error"=w4376:errorcluster, "output"=w4377:T14)  [unwired: 6 in, 1 out]
                n3406 = call <vilib>:"Clear Errors.vi"("error in (no error)"=w4376) -> ("error out"=w4375:errorcluster)  [unwired: 5 in, 1 out]
              }
            }
            n3407 = Unbundle By Name(w4360) -> ("LastCom"=→"LastCom":string, "Read Heave and Surge"=→"Read Humidity":string)
          }
        }
        n3408 = Divide(x="Surge PPR", y="Surge Pitch") -> (x/y=→"Surge Pulses/mm":dbl)
        n3409 = Unbundle By Name(w4335) -> ("Heave COM Status 2"=w4337:bool, "Heave COM Status"=w4336:bool, "Error Heave"=w4333:errorcluster, "Bytes at Heave Port"=→"Bytes at Humidity Port":dbl)
        n3410 = Unbundle By Name(w4333) -> ("status"=→"Humidity Port":bool)
        n3411 = Not(x=w4336) -> (.not. x?=w4321:bool)
        n3412 = local write "Error"(w4333) -> ()
        n3413 = Not(x=w4337) -> (.not. x?=w4322:bool)
        n3414 = local write "Instrument Status"(w4321) -> ()
        n3415 = local write "COM Status"(w4322) -> ()
        n3416 = local read "Quit"() -> (w4314:bool)
        n3417 = Select(t=enum16{"init", "MAIN", "Panel Close"}."Panel Close", s=w4314, f=enum16{"init", "MAIN", "Panel Close"}."MAIN") -> (s? t:f=w4313:enum16{"init", "MAIN", "Panel Close"})
      }
      frame "Panel Close" {
      }
      frame Default {
      }
    }
  }
  n3418 = while {
    stop <- w4418 stop-if-true
    n3419 = local read "Read Humidity"() -> (w4399:string)
    n3420 = call <vilib>:"High Resolution Polling Wait.vi"("seconds to wait"=0.1) -> ()  [unwired: 10 in, 1 out]
    n3421 = Spreadsheet String To Array(delimiter (Tab)=",", format string="", spreadsheet string=w4399, array type (2D Dbl)=string[] []) -> (array=w4413:string[])
    n3422 = for {
      tunnel: w4413 -> [w4423] mode=indexing
      tunnel: string[] ["STATE;", "SET;", "RH;", "T;", "AMB_RH;", "AMB_T;", "PUMP;", "FAN_IN;", "FAN_OUT;", "DEHUM;", "CURRENT;", "STALL;"] -> [w4422] mode=indexing
      tunnel: [w4421] -> w4412 mode=indexing
      n3423 = Match Pattern(string=w4423, regular expression=w4422) -> (after substring=w4421:string)  [unwired: 1 in, 3 out]
    }
    n3424 = Index Array(array=w4412) -> (element #1=→"STATE :":string, element #2=→"SET :":string, element #3=w4401:string, element #4=→"T :":string, element #5=w4398:string, element #6=→"AMB_T :":string, element #7=→"PUMP :":string, element #8=→"FAN_IN :":string, element #9=→"FAN_OUT :":string, element #10=→"DEHUM :":string, element #11=→"CURRENT :":string, element #12=→"STALL :":string)  [unwired: 12 in]
    "RH :" <- w4401
    "AMB_RH :" <- w4398
    n3425 = Fract/Exp String To Number(string=w4401) -> (number=w4393:dbl)  [unwired: 3 in, 1 out]
    n3426 = Fract/Exp String To Number(string=w4398) -> (number=w4397:dbl)  [unwired: 3 in, 1 out]
    n3427 = local write "Ambient Humidity :"(w4397) -> ()
    n3428 = Equal?(x=w4393, y=0.0) -> (x = y?=w4395:bool)
    n3429 = case shown="True" w4395 {
      tunnel: [w4419 w4420] -> w4394
      tunnel: w4393 -> [w4419 _]
      frame False {
        (unwired) 0.0
        "Humidity temp" <- w4419
      }
      frame True {
        n3430 = local read "Humidity temp"() -> (w4420:dbl)
      }
    }
    "RH Numeric:" <- w4394
    n3431 = local read "Quit"() -> (w4418:bool)
  }
  n3432 = disable-structure shown="Disabled" {
    frame Disabled {
      n3433 = while {
        tunnel: [w4657] -> _
        i -> [w4657]
        stop <- w4654 stop-if-true
        n3434 = local read "powstat"() -> (w4655:bool)
        n3435 = case shown="True" w4655 {
          frame False {
          }
          frame True {
            n3436 = local read "RUN"() -> (w4658:bool)
            n3437 = case shown="True" w4658 {
              frame False {
                w4688 = 65.0 ("y")
                n3438 = local read "Set Hz"() -> (w4716:dbl)
                n3439 = local read "NORMAL LOAD"() -> (w4717:dbl)
                n3440 = Multiply(x=w4716, y=60.0) -> (x*y=w4723:dbl)
                n3441 = Multiply(x=1.2 ("y"), y=0.949) -> (x*y=w4692:dbl)
                n3442 = Multiply(x=1.2 ("y"), y=0.8166) -> (x*y=w4696:dbl)
                n3443 = Multiply(x=1.2 ("y"), y=0.851) -> (x*y=w4691:dbl)
                n3444 = local read "FF 2"() -> (w4715:dbl)
                n3445 = Absolute Value(x=w4723) -> (abs(x)=w4721:dbl)
                n3446 = case shown="13.." w4715 {
                  tunnel: [1 2 3] -> w4713
                  frame 0..10, Default {
                    # "Normal"
                  }
                  frame 11, 12 {
                  }
                  frame 13.. {
                  }
                }
                "FF STATE" <- w4713
                n3447 = local read "TEMP"() -> (w4676:dbl)
                n3448 = local read item#-1() -> (w4690)
                n3449 = Less?(x=w4690, y=w4696) -> (x < y?=w4693:bool)
                n3450 = In Range and Coerce(upper limit=w4692, x=w4690, lower limit=w4691) -> (In Range?=w4694:bool)  [unwired: 1 out]
                n3451 = case shown="3601.." w4721 {
                  tunnel: [1 2 3] -> w4719
                  frame 0..3000, Default {
                    # "Normal"
                  }
                  frame 3001..3600 {
                  }
                  frame 3601.. {
                  }
                }
                n3452 = case shown="11.." w4717 {
                  tunnel: [1 3] -> w4718
                  frame 1..10, Default {
                  }
                  frame 11.. {
                  }
                }
                "NL STATE" <- w4718
                n3453 = Multiply(x=1.2 ("y"), y=0.95) -> (x*y=w4706:dbl)
                n3454 = Multiply(x=w4688, y=0.954) -> (x*y=w4680:dbl)
                n3455 = Or(x=w4693, y=w4694) -> (x .or. y?=w4695:bool)
                n3456 = Greater Or Equal?(x=w4690, y=w4706) -> (x >= y?=w4703:bool)
                n3457 = Multiply(x=w4688, y=0.99) -> (x*y=w4677:dbl)
                n3458 = Greater Or Equal?(x=w4676, y=w4677) -> (x >= y?=w4682:bool)
                n3459 = Greater Or Equal?(x=w4676, y=w4680) -> (x >= y?=w4679:bool)
                n3460 = case shown="0, 1, Default" w4690 {
                  tunnel: [1 3] -> w4707
                  frame 0, 1, Default {
                  }
                  frame 2.. {
                  }
                }
                n3461 = case shown="True" w4703 {
                  tunnel: [1 3] -> w4708
                  frame False {
                  }
                  frame True {
                  }
                }
                n3462 = case shown="True" w4695 {
                  tunnel: [1 2] -> w4709
                  frame False {
                  }
                  frame True {
                  }
                }
                n3463 = case shown="..0" w4676 {
                  tunnel: [2 3 3 1] -> w4683
                  frame 61, 62 {
                  }
                  frame 63.. {
                  }
                  frame ..0 {
                  }
                  frame 10..60, Default {
                  }
                }
                n3464 = case shown="True" w4682 {
                  tunnel: [1 3] -> w4684
                  frame False {
                  }
                  frame True {
                  }
                }
                n3465 = Number To Decimal String(number=w4719) -> (decimal integer string=w4720:string)  [unwired: 1 in]
                n3466 = case shown="True" w4679 {
                  tunnel: [1 2] -> w4685
                  frame False {
                  }
                  frame True {
                  }
                }
                n3467 = Number To Decimal String(number=1) -> (decimal integer string=→"Air temp":string)  [unwired: 1 in]
                n3468 = Number To Decimal String(number=w4713) -> (decimal integer string=→"ff_st":string)  [unwired: 1 in]
                n3469 = local write "sp_st"(w4720) -> ()
                n3470 = Number To Decimal String(number=w4718) -> (decimal integer string=→"nl_st":string)  [unwired: 1 in]
                n3471 = Build Array(w4683, w4684, w4685) -> (w4686:i32[])
                n3472 = Build Array(w4707, w4708, w4709) -> (w4710:i32[])
                n3473 = Array Max & Min(array=w4686) -> (max value=w4687:i32)  [unwired: 3 out]
                n3474 = Array Max & Min(array=w4710) -> (max value=w4711:i32)  [unwired: 3 out]
                n3475 = Number To Decimal String(number=w4687) -> (decimal integer string=w4675:string)  [unwired: 1 in]
                n3476 = Number To Decimal String(number=w4711) -> (decimal integer string=→"Stroke Ln 2":string)  [unwired: 1 in]
                n3477 = local write "temp_st"(w4675) -> ()
              }
              frame True {
                w4773 = 65.0 ("y")
                # "Healthy -1\nWarning -2\nError -3"
                n3478 = local read "TEMP"() -> (w4784:dbl)
                n3479 = local read "NORMAL LOAD"() -> (w4788:dbl)
                n3480 = local read "Set Hz"() -> (w4786:dbl)
                n3481 = Multiply(x=1.2 ("y"), y=0.949) -> (x*y=w4768:dbl)
                n3482 = Multiply(x=1.2 ("y"), y=0.8166) -> (x*y=w4764:dbl)
                n3483 = Multiply(x=1.2 ("y"), y=0.851) -> (x*y=w4769:dbl)
                n3484 = Multiply(x=w4773, y=0.954) -> (x*y=w4780:dbl)
                n3485 = Multiply(x=w4773, y=0.99) -> (x*y=w4783:dbl)
                n3486 = Greater Or Equal?(x=w4784, y=w4783) -> (x >= y?=w4778:bool)
                n3487 = Multiply(x=w4786, y=60.0) -> (x*y=w4792:dbl)
                n3488 = Greater Or Equal?(x=w4784, y=w4780) -> (x >= y?=w4781:bool)
                n3489 = local read "FF 2"() -> (w4787:dbl)
                n3490 = local read item#-1() -> (w4770)
                n3491 = Less?(x=w4770, y=w4764) -> (x < y?=w4767:bool)
                n3492 = In Range and Coerce(upper limit=w4768, x=w4770, lower limit=w4769) -> (In Range?=w4766:bool)  [unwired: 1 out]
                n3493 = Absolute Value(x=w4792) -> (abs(x)=w4790:dbl)
                n3494 = case shown="63.." w4784 {
                  tunnel: [2 3 3 1] -> w4777
                  frame 61, 62 {
                  }
                  frame 63.. {
                  }
                  frame ..0 {
                  }
                  frame 10..60, Default {
                  }
                }
                n3495 = case shown="True" w4778 {
                  tunnel: [1 3] -> w4776
                  frame False {
                  }
                  frame True {
                  }
                }
                n3496 = case shown="True" w4781 {
                  tunnel: [1 2] -> w4775
                  frame False {
                  }
                  frame True {
                  }
                }
                n3497 = Multiply(x=1.2 ("y"), y=0.95) -> (x*y=w4754:dbl)
                n3498 = case shown="1..10, Default" w4788 {
                  tunnel: [1 3] -> w4795
                  frame 1..10, Default {
                  }
                  frame 11.. {
                  }
                }
                n3499 = case shown="0..10, Default" w4787 {
                  tunnel: [1 2 3] -> w4794
                  frame 0..10, Default {
                  }
                  frame 11, 12 {
                  }
                  frame 13.. {
                  }
                }
                n3500 = case shown="3601.." w4790 {
                  tunnel: [1 2 3] -> w4789
                  frame 0..3000, Default {
                    # "Normal"
                  }
                  frame 3001..3600 {
                  }
                  frame 3601.. {
                  }
                }
                n3501 = Or(x=w4767, y=w4766) -> (x .or. y?=w4765:bool)
                n3502 = Greater Or Equal?(x=w4770, y=w4754) -> (x >= y?=w4757:bool)
                n3503 = case shown="0, 1, Default" w4770 {
                  tunnel: [1 3] -> w4753
                  frame 0, 1, Default {
                  }
                  frame 2.. {
                  }
                }
                n3504 = case shown="True" w4757 {
                  tunnel: [1 3] -> w4752
                  frame False {
                  }
                  frame True {
                  }
                }
                n3505 = case shown="True" w4765 {
                  tunnel: [1 2] -> w4751
                  frame False {
                  }
                  frame True {
                  }
                }
                n3506 = Build Array(w4777, w4776, w4775) -> (w4774:i32[])
                n3507 = Number To Decimal String(number=w4789) -> (decimal integer string=→"sp_st":string)  [unwired: 1 in]
                n3508 = Array Max & Min(array=w4774) -> (max value=w4771:i32)  [unwired: 3 out]
                "TEMP STATE" <- w4771
                n3509 = Number To Decimal String(number=w4795) -> (decimal integer string=w4798:string)  [unwired: 1 in]
                n3510 = Number To Decimal String(number=w4794) -> (decimal integer string=w4796:string)  [unwired: 1 in]
                n3511 = Number To Decimal String(number=w4771) -> (decimal integer string=→"temp_st":string)  [unwired: 1 in]
                n3512 = Build Array(w4753, w4752, w4751) -> (w4750:i32[])
                n3513 = local write "nl_st"(w4798) -> ()
                n3514 = local write "ff_st"(w4796) -> ()
                n3515 = Number To Decimal String(number=1) -> (decimal integer string=w4793:string)  [unwired: 1 in]
                n3516 = Array Max & Min(array=w4750) -> (max value=w4749:i32)  [unwired: 3 out]
                n3517 = local write "Air temp"(w4793) -> ()
                n3518 = Number To Decimal String(number=w4749) -> (decimal integer string=w4748:string)  [unwired: 1 in]
                n3519 = local write "Stroke Ln 2"(w4748) -> ()
              }
            }
            n3520 = local read "Stroke Ln 2"() -> (w4660:string)
            n3521 = local read "nl_st"() -> (w4666:string)
            n3522 = local read "ff_st"() -> (w4663:string)
            n3523 = local read "sp_st"() -> (w4664:string)
            n3524 = local read "temp_st"() -> (w4665:string)
            n3525 = local read "Air temp"() -> (w4659:string)
            n3526 = Replace Array Subset(array="in", new element #1=w4666, index #1=1 ("index"), new element #2=w4663, index #2=2 ("index"), new element #3=w4665, index #3=3 ("index"), new element #4=w4664, index #4=4 ("index"), new element #5=w4660, index #5=5 ("index"), new element #6=w4659, index #6=6 ("index"), new element #7="Sensor State" ("new element/subarray"), index #7=0 ("index")) -> (→"out":string[])
          }
        }
        n3527 = Wait (ms)(milliseconds to wait=u32 10) -> ()  [unwired: 1 out]
        n3528 = local read "Quit"() -> (w4654:bool)
      }
      n3529 = while {
        stop <- w4629 stop-if-true
        n3530 = local read "run replace"() -> (w4631:bool)
        n3531 = Wait (ms)(milliseconds to wait=u32 100) -> ()  [unwired: 1 out]
        n3532 = Equal?(x="FLAG 2", y=0.0) -> (x = y?=w4632:bool)
        n3533 = case shown="True" w4632 {
          frame False {
          }
          frame True {
            n3534 = local write "FLAG 2"(100.0 ("FLAG 2")) -> ()
            n3535 = call <vilib>:"Read Characters From File.vi"("file path (dialog if empty)"=path "C:/LAB-IQ-NXT/WO 2449 TT.sig", "convert eol? (no:F)"=FALSE ("append to file? (new file:F)")) -> ("character string"=w4635:string)  [unwired: 4 in, 3 out]
            n3536 = call <vilib>:"Read Characters From File.vi"("file path (dialog if empty)"=path "C:/LAB-IQ-NXT/WO 2449 TRH.sig", "convert eol? (no:F)"=FALSE ("append to file? (new file:F)")) -> ("character string"=w4636:string)  [unwired: 4 in, 3 out]
            n3537 = Decimal String To Number(string=w4635) -> (number=w4637:i32)  [unwired: 2 in, 1 out]
            n3538 = local write "Total No. of Tests"(w4637) -> ()
            n3539 = Decimal String To Number(string=w4636) -> (number=w4640:i32)  [unwired: 2 in, 1 out]
            n3540 = local write "SEN.RUN HRS"(w4640) -> ()
          }
        }
        n3541 = case shown="True" w4631 {
          frame False {
          }
          frame True {
            n3542 = Equal?(x="FLAG 4", y=0.0) -> (x = y?=w4644:bool)
            n3543 = case shown="False" w4644 {
              frame False {
                n3544 = Get Date/Time In Seconds() -> (seconds since 1Jan1904=w4650:timestamp)
                n3545 = local read "START 3"() -> (w4648:dbl)
                n3546 = To Double Precision Float(number=w4650) -> (double precision float=w4649:dbl)
                n3547 = Subtract(x=w4649, y=w4648) -> (x-y=→"SENSOR TIME":dbl)
              }
              frame True {
                n3548 = Get Date/Time In Seconds() -> (seconds since 1Jan1904=w4652:timestamp)
                n3549 = local write "FLAG 4"(100.0 ("FLAG")) -> ()
                n3550 = To Double Precision Float(number=w4652) -> (double precision float=→"START 3":dbl)
              }
            }
          }
        }
        n3551 = local read "Quit"() -> (w4629:bool)
      }
      n3552 = while {
        shift-right: [w4429] -> _
        shift-left: _ -> [w4430]
        tunnel: [w4425] -> _
        i -> [w4425]
        stop <- w4424 stop-if-true
        n3553 = Wait (ms)(milliseconds to wait=u32 50 ("Refresh Rate (ms)")) -> ()  [unwired: 1 out]
        n3554 = local read "Json End Flg"() -> (w4426:bool)
        n3555 = Not(x="Upld AR 2") -> ()  [unwired: 1 out]
        n3556 = local read "Upld AR 2"() -> (w4427:bool)
        n3557 = call "Elapsed Time9"("Time Target (s)"="Sen.Upload Rate (s)", "Reset"=FALSE, "Auto Reset"=TRUE) -> ("Time has Elapsed"=w4436:bool)  [unwired: 9 in, 7 out]
        n3558 = Or(x=w4436, y=w4426) -> (x .or. y?=w4432:bool)
        n3559 = case shown="True" w4432 {
          frame False {
          }
          frame True {
            w4528 = "\"SensorName\":\"" ("string")
            w4498 = " \"},{"
            w4523 = "\",\"SensorState\":\""
            w4525 = "\",\"SensorModelNumber\":\"" ("string")
            w4524 = "\",\"SensorRuntimeHours\":\"" ("string")
            n3560 = local read "model num"() -> (w4522:string[])
            n3561 = local read "Sensor name"() -> (w4541:string[])
            n3562 = local read "run"() -> (w4512:string[])
            n3563 = local read "SENSOR TIME"() -> (w4468:dbl)
            n3564 = local read "out"() -> (w4461:string[])
            n3565 = local read "Total No. of Tests"() -> (w4466:dbl)
            n3566 = Select(t=60.0, s="Run test 3", f=3600.0) -> (s? t:f=w4476:dbl)
            n3567 = Index Array(array=w4522, index #1=1 ("index")) -> (element #1=w4521:string, element #2=w4520:string, element #3=w4519:string, element #4=w4518:string, element #5=w4517:string, element #6=w4516:string)  [unwired: 5 in]
            n3568 = Index Array(array=w4512, index #1=1 ("index")) -> (element #1=w4511:string, element #2=w4510:string, element #3=w4509:string, element #4=w4508:string, element #5=w4507:string, element #6=w4506:string)  [unwired: 5 in]
            n3569 = Index Array(array=w4541, index #1=1 ("index")) -> (element #1=w4540:string, element #2=w4539:string, element #3=w4538:string, element #4=w4537:string, element #5=w4527:string, element #6=w4526:string)  [unwired: 5 in]
            n3570 = Index Array(array=w4461, index #1=1 ("index")) -> (element #1=w4493:string, element #2=w4492:string, element #3=w4491:string, element #4=w4490:string, element #5=w4489:string, element #6=w4488:string)  [unwired: 5 in]
            n3571 = local read "SEN.RUN HRS"() -> (w4464:dbl)
            n3572 = Divide(x=w4468, y=w4476) -> (x/y=w4475:dbl)
            n3573 = Increment(x=w4475) -> (x+1=w4471:dbl)
            n3574 = Number To Decimal String(number=w4471) -> (decimal integer string=→"run hrs":string)  [unwired: 1 in]
            n3575 = Divide(x=w4464, y=3600.0 ("f")) -> (x/y=w4459:dbl)
            n3576 = Round To Nearest(number=w4459) -> (nearest integer value=w4457:dbl)
            n3577 = Number To Decimal String(number=w4457) -> (decimal integer string=w4458:string)  [unwired: 1 in]
            n3578 = Number To Decimal String(number=w4466) -> (decimal integer string=w4467:string)  [unwired: 1 in]
            n3579 = local read "Model No"() -> (w4472:string)
            n3580 = local read "UUID"() -> (w4567:string)
            n3581 = local read "Serial No"() -> (w4571:string)
            n3582 = local read "Secret Key"() -> (w4572:string)
            n3583 = Concatenate Strings("\",\"MachineSerialNumber\":\"" ("string"), w4571) -> (w4575:string)
            n3584 = Concatenate Strings("\",\"ModelNumber\":\"" ("string"), w4472) -> (w4473:string)
            n3585 = Concatenate Strings("\",\"MachineRuntimeHours\":\"" ("string"), w4458) -> (w4576:string)
            n3586 = Concatenate Strings("\",\"MachineRuntimeCycles\":\"", w4467) -> (w4569:string)
            n3587 = Concatenate Strings(w4525, w4521) -> (w4555:string)
            n3588 = Concatenate Strings(w4524, w4511) -> (w4556:string)
            n3589 = Concatenate Strings(w4523, w4493) -> (w4554:string)
            n3590 = Concatenate Strings(w4575, w4473, w4576, w4569) -> (w4578:string)
            n3591 = Concatenate Strings(w4525, w4520) -> (w4552:string)
